vi "Update UI.vi"(8 "error in (no error)":errorcluster, 11 "SE UI cluster in":T1={"Node Ptr"=18446744073709551615, "Add"=refnum, "Remove"=refnum, "Registers ListBox"=refnum} {"Node Ptr" format="%.0x"}) -> (0 "error out":errorcluster, 3 "SE UI cluster out":T1={"Node Ptr"=18446744073709551615, "Add"=refnum, "Remove"=refnum, "Registers ListBox"=refnum} {"Node Ptr" format="%.0x"})   [LabVIEW 2020, in "FPGA Addon System Explorer.lvlib"]
uses:
  FPGA Addon System Explorer.lvlib
  Types/SE UI Cluster.ctl
  <vilib>/NI VeriStand/Custom Device API/Custom Device Item Ref.ctl
  <vilib>/NI VeriStand/Custom Device API/Custom Device API.lvlib
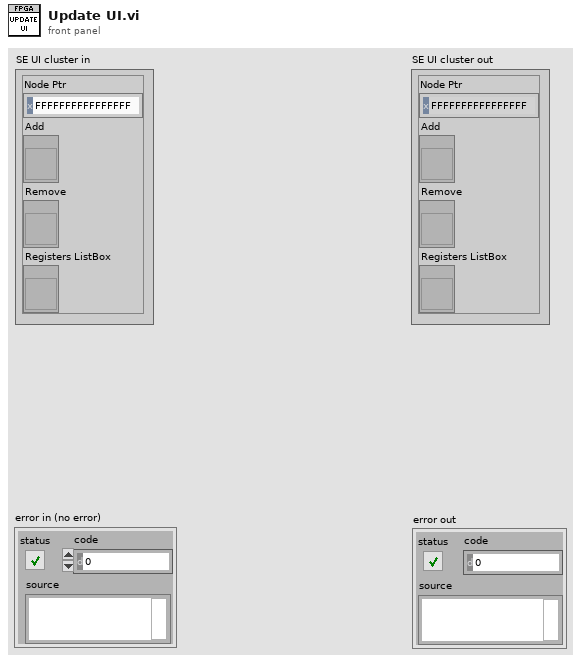
[diagram p1: front panel]
types:
  T1 = typedef "FPGA Addon System Explorer.lvlib/SE UI Cluster.ctl" = cluster{"Node Ptr":T2, "Add":refnum<vi>, "Remove":refnum<vi>, "Registers ListBox":refnum<vi>}
  T2 = typedef "Custom Device API.lvlib/Custom Device Item Ref.ctl" = u64
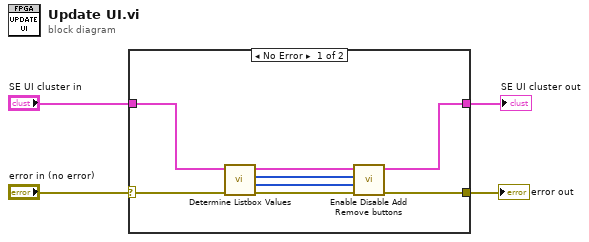
[diagram p0: block diagram]
diagram:
  n1 = case shown="No Error" "error in (no error)" {
    selector: "error in (no error)" -> [w5 w13]
    tunnel: [w12 w13] -> w4
    tunnel: "SE UI cluster in" -> [w11 w14]
    tunnel: [w6 w14] -> w2
    frame No Error {
      n2 = call "Determine Listbox Values.vi"("error in (no error)"=w5, "SE UI cluster in"=w11) -> ("error out"=w10:errorcluster, "Not imported item Indexes"=w7:i32[], "Selected item indexes"=w8:i32[], "SE UI cluster out"=w9:T1)  [unwired: 6 in]
      n3 = call "Enable Disable Add Remove buttons.vi"("error in (no error)"=w10, "Not imported item Indexes"=w7, "Selected item indexes"=w8, "SE UI cluster in"=w9) -> ("error out"=w12:errorcluster, "SE UI cluster out"=w6:T1)  [unwired: 6 in]
    }
    frame Error {
    }
  }
  "error out" <- w4
  "SE UI cluster out" <- w2
